vi "CAN write.vi"(8 "error in":errorcluster, 9 "Data":u8[](array[numeric]), 10 "COB-ID":u32 format="%.0x", 11 "CANopen in":refnum<class "CANopen.lvclass">) -> (0 "error out":errorcluster, 3 "CANopen out":refnum<class "CANopen.lvclass">)   [LabVIEW 2026, in "canopen_.lvlib" / "CANopen.lvclass"]
doc: "Sends a bunch of data to a specific COB-ID."
uses:
  CANopen.lvclass
  CANopen.lvclass/CANopen.ctl
  HAL/HAL/Protocols/ICAN/ICAN.lvclass
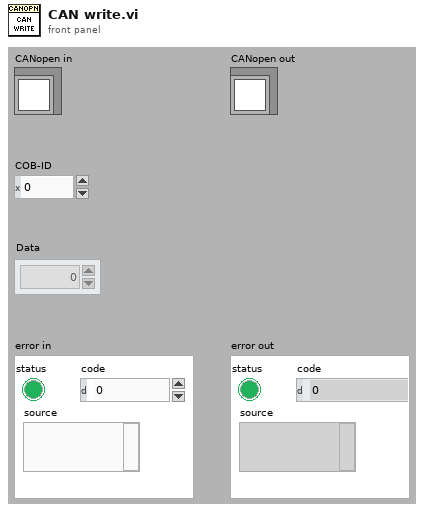
[diagram p1: front panel]
types:
  T1 = cluster{"ID":u32, "MSG type":u8, "DLC":u8, "DATA":u8[]}
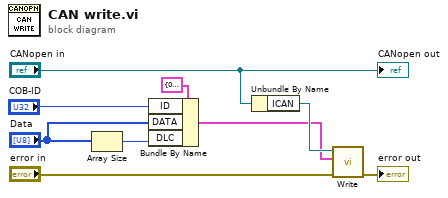
[diagram p0: block diagram]
diagram:
  n1 = Array Size(array="Data") -> (size(s)=w7:i32)
  n2 = Bundle By Name(cluster=T1 {"ID"=0, "MSG type"=0, "DLC"=0, "DATA"=[]} ("CAN Message"), "ID"="COB-ID", "DATA"="Data", "DLC"=w7) -> (w1:T1)
  n3 = Unbundle By Name("CANopen in") -> ("ICAN"=w9:refnum<class "ICAN.lvclass">)
  n4 = call-dynamic "Write.vi"("error in"="error in", "CAN Message"=w1, "ICAN in"=w9) -> ("error out"=→"error out":errorcluster)  [unwired: 7 in, 1 out]
  "CANopen out" <- "CANopen in"
